vi "sendErrorLog.vi"(8 "error in (no error)":errorcluster, 11 "message out":T1) -> (0 "error out":errorcluster)   [LabVIEW 2017, in "loggingModule.lvlib"]
doc: "This VI passes along error information to the loggin module for logging as a high priority message."
uses:
  loggingModule.lvlib
  ErrorMonitor/Queue/TypeDefs/message.ctl
  Queue/TypeDefs/queueFGVState.ctl
  Queue/TypeDefs/message.ctl
  ErrorMonitor/ErrorMonitor.lvlib
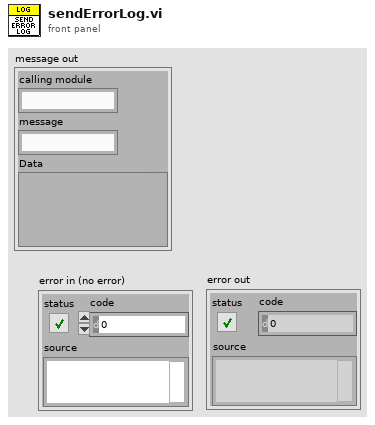
[diagram p1: front panel]
types:
  T1 = typedef "ErrorMonitor.lvlib/message.ctl" = cluster{"calling module":string, "message":string, "Data":variant}
  T2 = typedef "loggingModule.lvlib/message.ctl" = cluster{"calling module":string, "message":string, "data":variant}
  T3 = typedef "loggingModule.lvlib/queueFGVState.ctl" = enum16{"obtain", "enqueue low priority", "enqueue high priority", "dequeue", "release"}
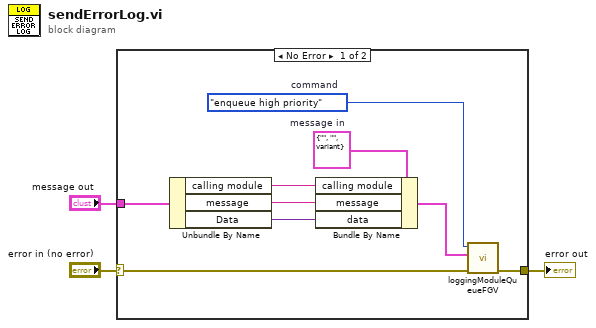
[diagram p0: block diagram]
diagram:
  n1 = case shown="No Error" "error in (no error)" {
    selector: "error in (no error)" -> [w12 w13]
    tunnel: [w11 w13] -> w2
    tunnel: "message out" -> [w7 _]
    frame No Error {
      w9 = T2 {"calling module"="", "message"="", "data"=variant}  # message in
      w10 = queueFGVState."enqueue high priority"  # command
      n2 = Unbundle By Name(w7) -> ("calling module"=w6:string, "message"=w5:string, "Data"=w4:variant)
      n3 = Bundle By Name(cluster=w9, "calling module"=w6, "message"=w5, "data"=w4) -> (w8:T2)
      n4 = call "loggingModuleQueueFGV.vi"("error in (no error)"=w12, "message in"=w8, "command"=w10) -> ("error out"=w11:errorcluster)  [unwired: 7 in, 1 out]
    }
    frame Error {
    }
  }
  "error out" <- w2
